vi "AlazarDSPGenerateWindowFunction.vi"(0 "Handle":u64, 1 "Window Type":u32(ring)=4 items=["None", "Hanning", "Hamming", "Blackman", "Blackman-Harris", "Bartlett"], 2 "window":sgl[](array[numeric]), 3 "WindowLength_samples":u32, 4 "PaddingLength_samples":u32, 5 "error in (no error)":errorcluster) -> (14 "Handle":u64, 15 "window":sgl[](array[numeric]), 18 "Return Code":u32, 19 "error out":errorcluster)   [LabVIEW 2018]
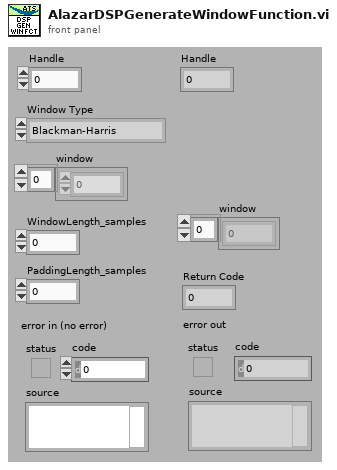
[diagram p1: front panel]
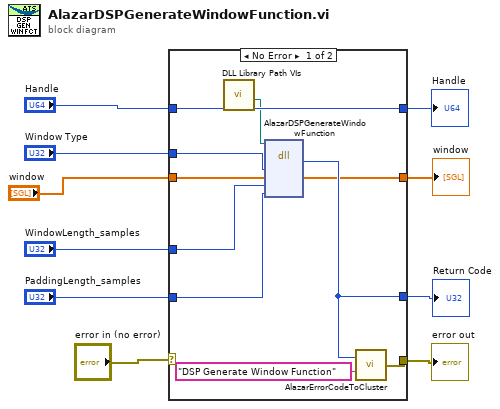
[diagram p0: block diagram]
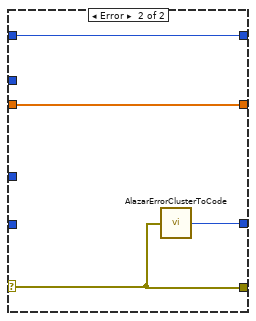
[diagram p2: hidden frame]
diagram:
  n1 = case shown="No Error" "error in (no error)" {
    selector: "error in (no error)" -> [_ w24]
    tunnel: [w18 w24] -> w9
    tunnel: [w20 w23] -> w8
    tunnel: "Handle" -> [w13 w22]
    tunnel: [w13 w22] -> w6
    tunnel: "window" -> [w17 w21]
    tunnel: "WindowLength_samples" -> [w16 _]
    tunnel: "PaddingLength_samples" -> [w15 _]
    tunnel: [w14 w21] -> w2
    tunnel: "Window Type" -> [w12 _]
    frame No Error {
      n2 = call "DLL Library Path VIs.vi"() -> ("Alazar"=w11:path)  [unwired: 5 in, 6 out]
      n3 = dll-call lib="C:/Project/SerialSectOCT - FFT GPU/SerialSectOCT/Labview Software/DLL/ATSApi.dll" fn="AlazarDSPGenerateWindowFunction"(path in=w11, "windowType"=w12, "window"=w17, "windowLength_samples"=w16, "paddingLength_samples"=w15) -> ("return type"=w20:u32, "window"=w14:sgl[])  [unwired: 5 in, 2 out]
      n4 = call "AlazarErrorCodeToCluster.vi"("Message"="DSP Generate Window Function", "Error Code"=w20) -> ("error out"=w18:errorcluster)
    }
    frame Error {
      n5 = call "AlazarErrorClusterToCode.vi"("error in (no error)"=w24) -> ("Error Code"=w23:u32)
    }
  }
  "Handle" <- w6
  "error out" <- w9
  "Return Code" <- w8
  "window" <- w2
